vi "Initialize AI.vi"(8 "error in (no error)":errorcluster, 9 "AI Setting":T1={"Physical Channel"=["6363/ai0", "6363/ai1", "6363/ai2"], "Name to assign"=[], "input terminal configuration"=enum."RSE", "minimum value"=0.0, "maximum value"=10.0, "units"=enum."Volts", "custom scale name"="", "sample mode"=enum."Finite Samples", "rate"=5000.0, "samples per channel"=1000} {"rate" format="%#_13g"; "maximum value" format="%#_13g"; "minimum value" format="%#_13g"}, 10 "DAQ Type":enum16{"Hardware", "Simulation"}(ring), 11 "Abstract in":refnum<class "Abstract.lvclass">) -> (0 "error out":errorcluster, 3 "Abstract out":refnum<class "Abstract.lvclass">)   [LabVIEW 2021, in "DAQ Hardware.lvlib" / "Abstract.lvclass"]
uses:
  Abstract.lvclass
  User Interface/AI Channel Setting.ctl
  DAQ Hardware.lvlib
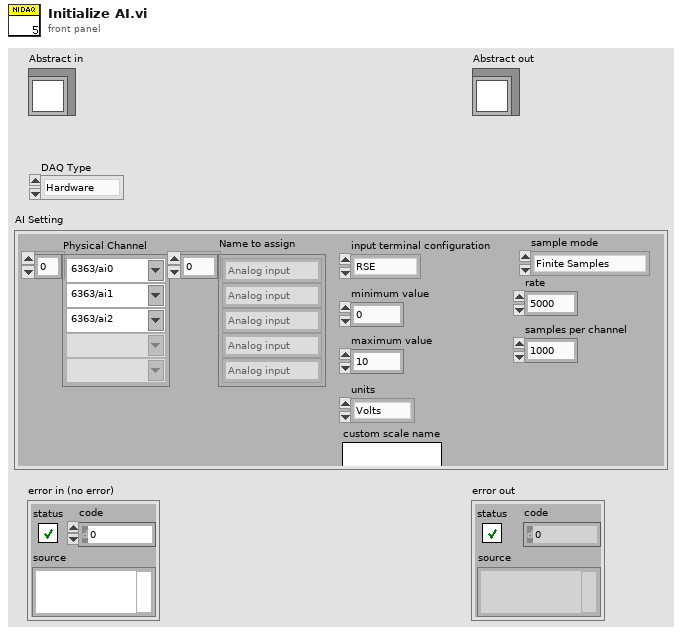
[diagram p1: front panel]
types:
  T1 = typedef "DAQ Hardware.lvlib/AI Channel Setting.ctl" = cluster{"Physical Channel":string[], "Name to assign":string[], "input terminal configuration":enum16{"RSE", "NRSE", "Differential"}, "minimum value":dbl, "maximum value":dbl, "units":enum16{"Volts"}, "custom scale name":string, "sample mode":enum16{"Finite Samples", "Continuous Samples", "Hardware Timed Single Point"}, "rate":dbl, "samples per channel":i32}
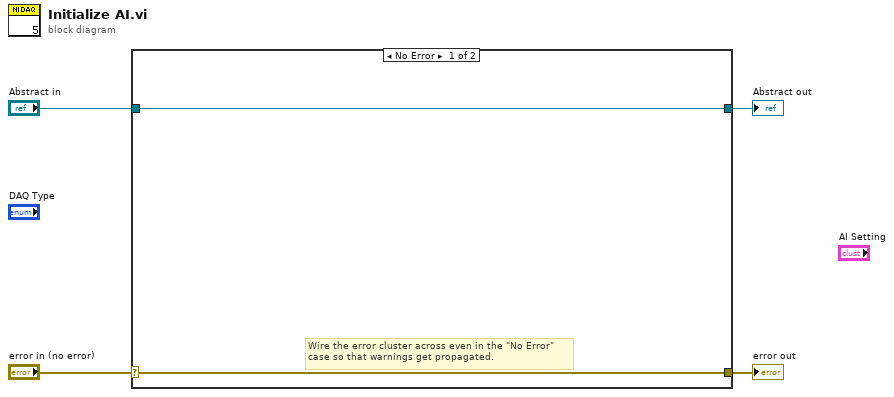
[diagram p0: block diagram]
diagram:
  n1 = case shown="No Error" "error in (no error)" {
    selector: "error in (no error)" -> [w5 w8]
    tunnel: [w5 w8] -> w3
    tunnel: [w6 w7] -> w1
    tunnel: "Abstract in" -> [w6 w7]
    frame No Error {
      # "Wire the error cluster across even in the \"No Error\"\ncase so that warnings get propagated."
    }
    frame Error {
    }
  }
  "error out" <- w3
  "Abstract out" <- w1
